vi "InitialUninstall.vi"(2 "unIndex":bool[](array[boolean]), 3 "Trip Status":refnum<vi>) -> ()   [LabVIEW 2015]
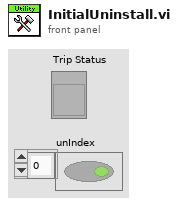
[diagram p1: front panel]
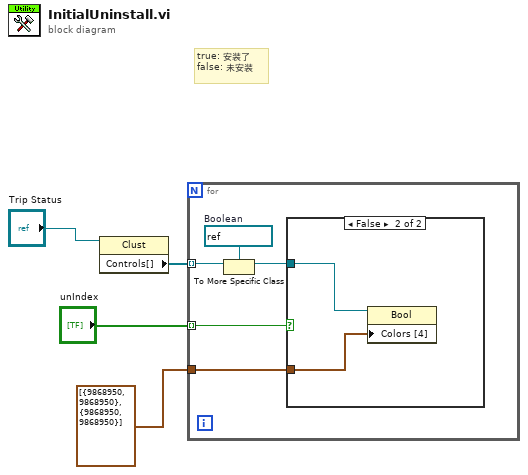
[diagram p0: block diagram]
diagram:
  # "true: 安装了\nfalse: 未安装"
  n1 = property class="Clust"(reference="Trip Status") -> ("Controls[]"=w3:refnum<vi>[])  [unwired: 1 in, 2 out]
  n2 = for {
    tunnel: w3 -> [w9] mode=indexing
    tunnel: cluster{u32, u32}[] [{9868950, 9868950}, {9868950, 9868950}] ("Array") -> [w6]
    tunnel: "unIndex" -> [w5] mode=indexing
    w8 = refnum<vi> refnum  # Boolean
    n3 = To More Specific Class(target class=w8, reference=w9) -> (specific class reference=w7:refnum<vi>)  [unwired: 1 in, 1 out]
    n4 = case shown="False" w5 {
      tunnel: w7 -> [_ w11]
      tunnel: w6 -> [_ w10]
      frame True {
      }
      frame False {
        n5 = property class="Bool"(reference=w11, "Colors [4]"=w10) -> ()  [unwired: 1 in, 2 out]
      }
    }
  }
